vi "ModifyTileCode.vi"(8 "replace_color":fxp<+,3,3>, 9 "color_to_replace":fxp<+,3,3>=7.0, 10 "rotation":u8, 11 "tilenumber":u8) -> (3 "TileCode":u16)   [LabVIEW 2019, in "RT_Game.lvlib" / "Game.lvclass"]
uses:
  Game.lvclass
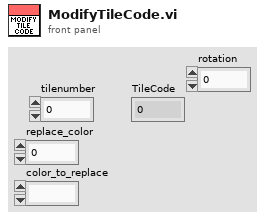
[diagram p1: front panel]
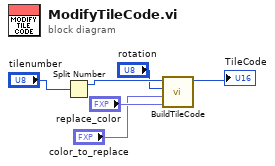
[diagram p0: block diagram]
diagram:
  n1 = Split Number(x="tilenumber") -> (hi(x)=w4:u8)  [unwired: 1 out]
  n2 = call "BuildTileCode.vi"("replace_color"="replace_color", "color_to_replace"="color_to_replace", "rotation"="rotation", "tilenumber"=w4) -> ("TileCode"=→"TileCode":u16)  [unwired: 7 in]
